vi "Disconnect.vi"(8 "error in":errorcluster, 11 "IMG_SRC in":refnum<class "IMG_SRC.lvclass">) -> (0 "error out":errorcluster, 3 "IMG_SRC out":refnum<class "IMG_SRC.lvclass">)   [LabVIEW 2018, in "IMG_SRC.lvlib" / "IMG_SRC.lvclass"]
uses:
  IMG_SRC.lvclass
  IMG_SRC.lvclass/IMG_SRC.ctl
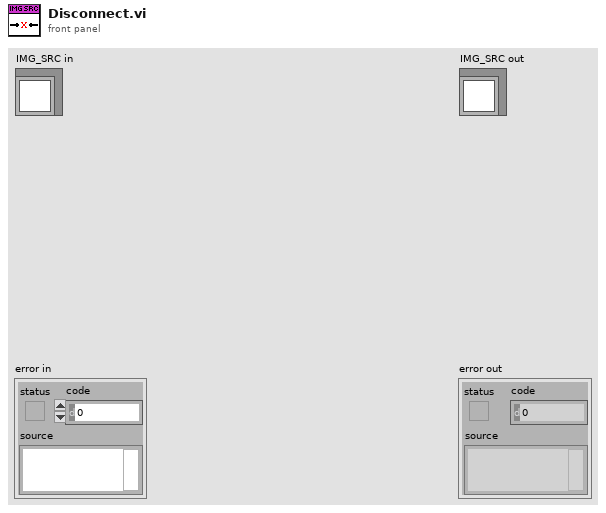
[diagram p1: front panel]
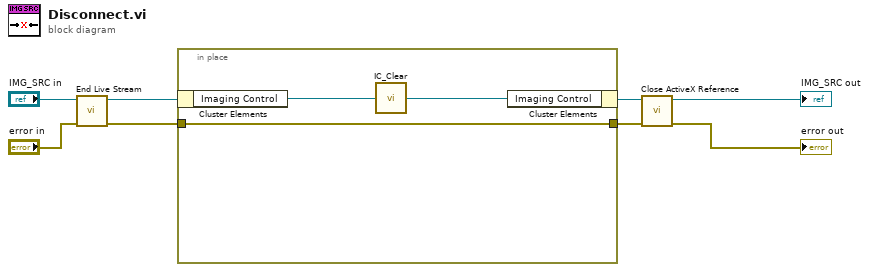
[diagram p0: block diagram]
diagram:
  n1 = call "End Live Stream.vi"("error in"="error in", "IMG_SRC in"="IMG_SRC in") -> ("error out"=w2:errorcluster, "IMG_SRC out"=w1:refnum<class "IMG_SRC.lvclass">)  [unwired: 8 in]
  n2 = in-place {
    in-place-border: [w9] -> w7
    in-place-border: w2 -> [w9]
    n3 = in-place-cluster #1(w1) -> ("Imaging Control"=w11:refnum<k7>)
    n4 = call <userlib>:"IC_Clear.vi"("ICImagingControl 2"=w11) -> ("ICImagingControl"=w10:refnum<k7>)
    n5 = in-place-cluster #1("Imaging Control"=w10) -> (w8:refnum<class "IMG_SRC.lvclass">)
  }
  n6 = call "Close ActiveX Reference.vi"("error in"=w7, "IMG_SRC in"=w8) -> ("error out"=→"error out":errorcluster, "IMG_SRC out"=→"IMG_SRC out":refnum<class "IMG_SRC.lvclass">)  [unwired: 8 in]
